vi "compressor.vi"() -> (0 "On/Off":bool=TRUE, 1 "Charging":bool, 2 "Full":bool)   [LabVIEW 2015]
uses:
  <vilib>/Rock Robotics/Network Tables/NT Read Boolean Array.vi
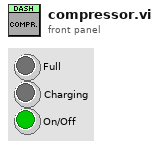
[diagram p1: front panel]
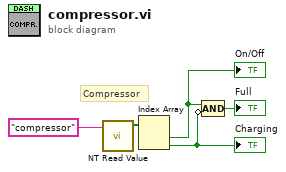
[diagram p0: block diagram]
diagram:
  # "Compressor"
  n1 = call-poly <vilib>:"NT Read Value.vi"("Name"="compressor") -> ("Boolean Array"=w1:bool[])  [unwired: 9 in, 1 out]
  n2 = Index Array(array=w1) -> (element #1=w3:bool, element #2=w2:bool)  [unwired: 2 in]
  "Charging" <- w2
  "On/Off" <- w3
  n3 = Compound Arithmetic op=AND(w3, invert w2) -> (→"Full":bool)
